vi "Event FGV.vi"(8 "error in (no error)":errorcluster, 11 "FGV Action":T1) -> (0 "error out":errorcluster, 3 "Event Data":refnum<user-event>)   [LabVIEW 2020, in "User Event.lvlib"]
doc: "For name actions"
uses:
  User Event.lvlib
  FGV Action.ctl
  Event Data.ctl
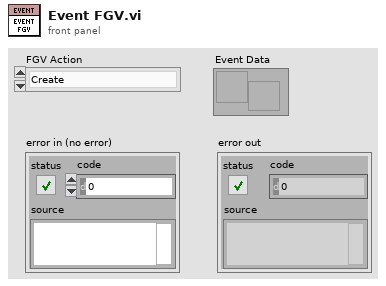
[diagram p1: front panel]
types:
  T1 = typedef "User Event.lvlib/FGV Action.ctl" = enum16{"Create", "Get", "Destroy"}
  T2 = typedef "User Event.lvlib/Event Data.ctl" = enum16{"Exit Program"}
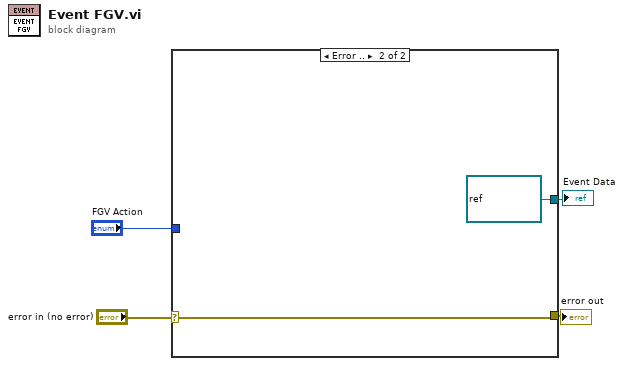
[diagram p0: block diagram]
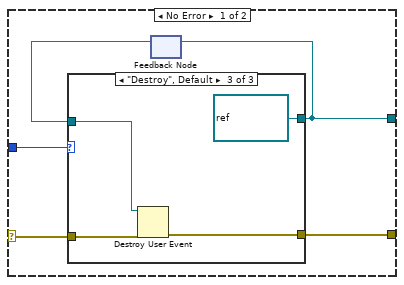
[diagram p2: hidden frame]
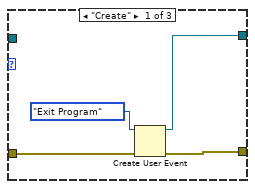
[diagram p3: hidden frame]
diagram:
  n1 = case shown="Error .." "error in (no error)" {
    selector: "error in (no error)" -> [w8 w21]
    tunnel: "FGV Action" -> [w9 _]
    tunnel: [w6 w21] -> w2
    tunnel: [w5 w20] -> w1
    frame No Error {
      n2 = feedback #1() -> (w7:refnum<user-event>)  [unwired: 1 in]
      n3 = case shown="\"Destroy\", Default" w9 {
        tunnel: w8 -> [w13 w14 w18]
        tunnel: [w11 w14 w16] -> w6
        tunnel: [w10 w15 w17] -> w5
        tunnel: w7 -> [_ w15 w19]
        frame "Create" {
          n4 = Create User Event(user event datatype=Event_Data."Exit Program" ("Event Data"), error in=w13) -> (user event=w10:refnum<user-event>, error out=w11:errorcluster)
        }
        frame "Get" {
        }
        frame "Destroy", Default {
          w17 = refnum<user-event> refnum items=["Exit Program"] ("Event Data")
          n5 = Destroy User Event(user event=w19, error in=w18) -> (error out=w16:errorcluster)
        }
      }
      n6 = feedback-in #1(w5) -> ()
    }
    frame Error {
      w20 = refnum<user-event> refnum items=["Exit Program"] ("Event Data")
    }
  }
  "error out" <- w2
  "Event Data" <- w1
